vi "Check for Timeout.vi"(0 "error message":string, 5 "complete?":bool, 7 "start time":timestamp, 11 "error in":errorcluster) -> (15 "error out":errorcluster)   [LabVIEW 2020]
doc: "Returns an error if timeout has occurred.\n\n<B>Input Parameters</B>\n\n<B>Error Message</B> is the message string to report in the error message.\n\n<B>Complete?</B> specifies if the loop has completed, in which case timeout is not checked.\n\n<B>Start Time</B> is the start time to check against to determine if timeout has occurred.\n\n<B>error in</B> describes error conditions that occur before this node runs. This input provides standard error in functionality.\n\n<B>Output Parameters</B>\n\n<B>error out</B> contains error information. This output provides standard error out functionality."
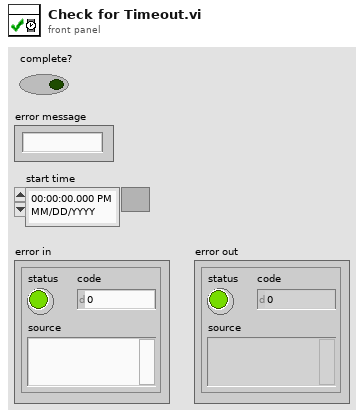
[diagram p1: front panel]
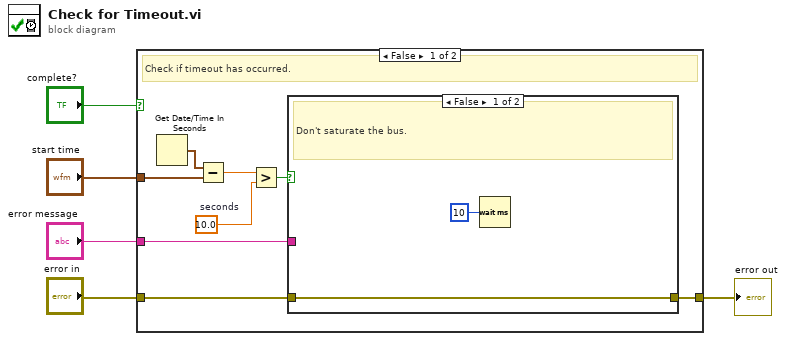
[diagram p0: block diagram]
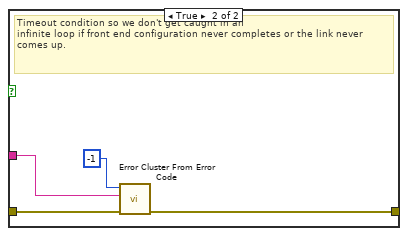
[diagram p2: hidden frame]
diagram:
  n1 = case shown="False" "complete?" {
    tunnel: "error in" -> [w13 w20]
    tunnel: "start time" -> [w9 _]
    tunnel: [w7 w20] -> w1
    tunnel: "error message" -> [w6 _]
    frame False {
      w11 = 10.0  # seconds
      # "Check if timeout has occurred."
      n2 = Get Date/Time In Seconds() -> (seconds since 1Jan1904=w8:timestamp)
      n3 = Subtract(x=w8, y=w9) -> (x-y=w10:dbl)
      n4 = Greater?(x=w10, y=w11) -> (0:w12:bool)
      n5 = case shown="False" w12 {
        tunnel: w13 -> [w15 w19]
        tunnel: [w15 w18] -> w7
        tunnel: w6 -> [_ w16]
        frame False {
          # "Don't saturate the bus."
          n6 = Wait (ms)(milliseconds to wait=u32 10) -> ()  [unwired: 1 out]
        }
        frame True {
          # "Timeout condition so we don't get caught in an\ninfinite loop if front end configuration never completes or the link never comes up."
          n7 = call <vilib>:"Error Cluster From Error Code.vi"("error in (no error)"=w19, "error message (\"\")"=w16, "error code (0)"=-1) -> ("error out"=w18:errorcluster)  [unwired: 6 in]
        }
      }
    }
    frame True {
      # "No need to check timeout as the condition we desired has occurred."
    }
  }
  "error out" <- w1
